vi "SetOffsets.vi"(0 "reference":refnum<class "ClassRelationshipEdge.lvclass">, 1 "startConnectionOffset":cluster{"x":i32, "y":i32}, 2 "MidLineOffset":cluster{"x":i32, "y":i32}, 3 "endConnectionOffset":cluster{"x":i32, "y":i32}, 5 "error in (no error)":errorcluster) -> (14 "reference out":refnum<class "ClassRelationshipEdge.lvclass">, 19 "error out":errorcluster)   [LabVIEW 2020, in "ClassRelationshipEdge.lvclass"]
uses:
  <resource>/Framework/Providers/Open_GDS/UML/ClassRelationshipEdge_class/ClassRelationshipEdge.lvclass
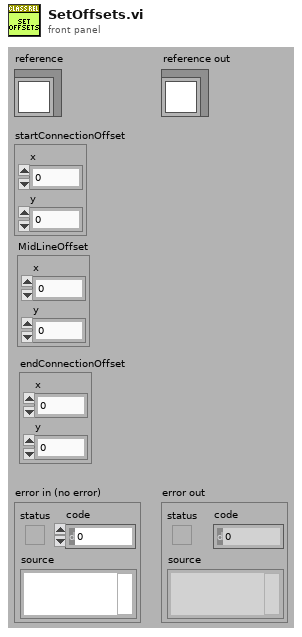
[diagram p1: front panel]
types:
  T1 = typedef "ClassRelationshipEdge.lvclass/ObjectAttributes.ctl" = cluster{"bentStyleRef":refnum<class "BentStyle.lvclass">, "startConnectionOffset":cluster{"x":i32, "y":i32}, "endConnectionOffset":cluster{"x":i32, "y":i32}, "MidLineOffset":cluster{"x":i32, "y":i32}, "DepClass":T2}
  T2 = typedef "ReversedEngineering_ViDependencyDetailsType.ctl" = cluster{"ThisVIs/Ctls":path[], "Dependent_VIs/Ctls":path[]}
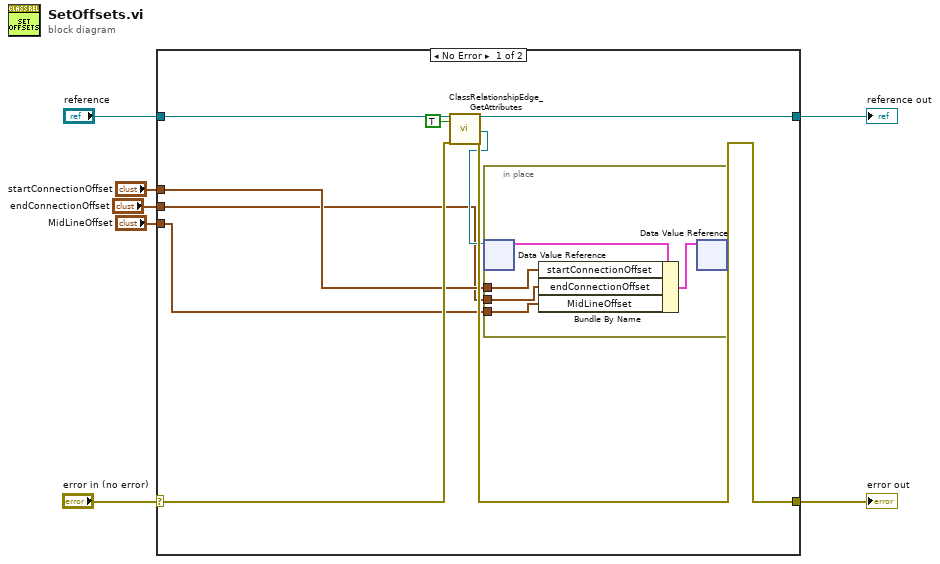
[diagram p0: block diagram]
diagram:
  n1 = case shown="No Error" "error in (no error)" {
    selector: "error in (no error)" -> [w16 w22]
    tunnel: "reference" -> [w15 w23]
    tunnel: [w14 w22] -> w5
    tunnel: [w13 w23] -> w4
    tunnel: "startConnectionOffset" -> [w10 _]
    tunnel: "endConnectionOffset" -> [w9 _]
    tunnel: "MidLineOffset" -> [w8 _]
    frame No Error {
      n2 = call <resource>:"ClassRelationshipEdge_GetAttributes.vi"("reference in"=w15, "OnlyGetDvrReference(False)"=TRUE, "error in (no error)"=w16) -> ("reference out"=w13:refnum<class "ClassRelationshipEdge.lvclass">, "DataRef"=w11:refnum<data-value>, "error out"=w14:errorcluster)  [unwired: 13 in, 1 out]
      n3 = in-place {
        in-place-border: w10 -> [w20]
        in-place-border: w9 -> [w19]
        in-place-border: w8 -> [w18]
        n4 = in-place-dvr #1(w11) -> (w21:T1)  [unwired: 1 out]
        n5 = Bundle By Name(cluster=w21, "startConnectionOffset"=w20, "endConnectionOffset"=w19, "MidLineOffset"=w18) -> (w17:T1)
        n6 = in-place-dvr #1(w17) -> ()  [unwired: 2 out]
      }
    }
    frame Error {
    }
  }
  "reference out" <- w4
  "error out" <- w5
